vi "Auto Filenames Postprocessing.vi"(8 "Fehler (Eingang)":errorcluster, 9 "active postprocessing index":i32) -> (0 "Fehler (Ausgang)":errorcluster, 1 "active reprocessing index out":i32, 2 "postprocess LIN Filename":string, 3 "postprocess LIN Pfad":path)   [LabVIEW 2020, in "Linearisierung v2.lvlib" / "SpanEinstellungen.lvlib"]
uses:
  SpanEinstellungen.lvlib
  Aktion FGV Post Processing.ctl
  Allgemein/allgemeine Sub-VIs.lvlib
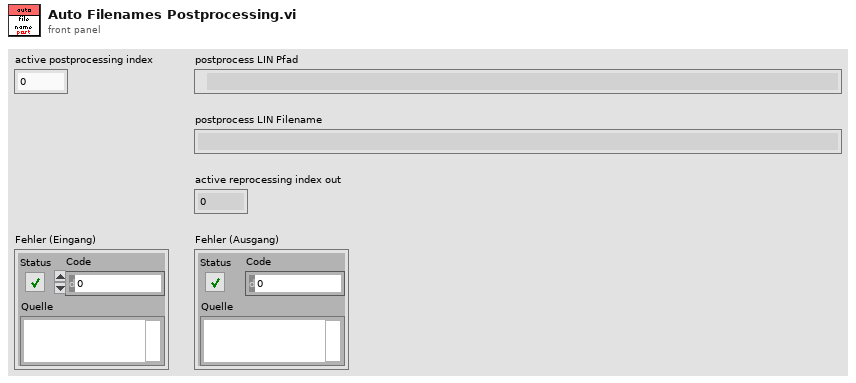
[diagram p1: front panel]
types:
  T1 = typedef "Linearisierung v2.lvlib/SpanEinstellungen.lvlib/Aktion FGV Post Processing.ctl" = enum16{"lesen", "set ref", "init", "reset", "enable", "disable", "filenames", "active", "comp", "filename index", "next", "first", "abort", "show"}
  T2 = typedef "Pfad-Eingabefeld.ctl" = path
  T3 = cluster{"active SPAN Idx":i32, "Pfad .LIN Datei":T2}[]
  T4 = cluster{"active SPAN Idx":i32, "Pfad .LIN Datei":T2}
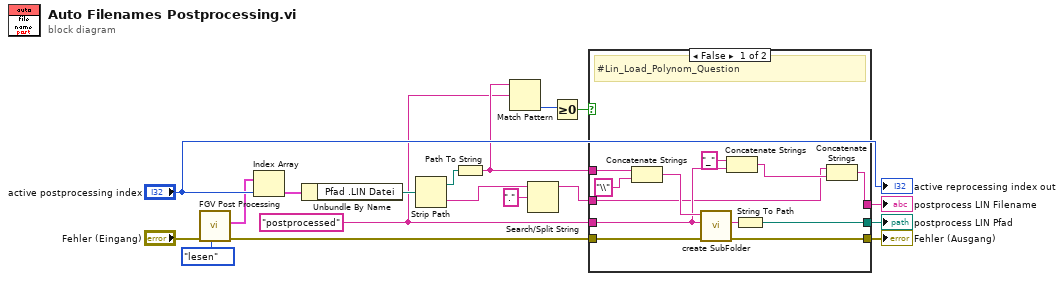
[diagram p0: block diagram]
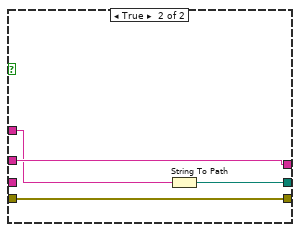
[diagram p2: hidden frame]
diagram:
  w6 = "postprocessed" ("String")
  n1 = call "FGV Post Processing.vi"("Aktion"=Aktion_FGV_Post_Processing."lesen", "error in (no error)"="Fehler (Eingang)") -> ("error out"=w9:errorcluster, "filenemas Cluster Array"=w15:T3)  [unwired: 6 in, 2 out]
  n2 = Index Array(array=w15, index="active postprocessing index") -> (element=w14:T4)
  n3 = Unbundle By Name(w14) -> ("Pfad .LIN Datei"=w13:T2)
  n4 = Strip Path(path=w13) -> (stripped path=w12:path, name=w2:string)
  n5 = Path To String(path=w12) -> (string=w7:string)
  n6 = Match Pattern(string=w7, regular expression=w6) -> (offset past match=w5:i32)  [unwired: 1 in, 3 out]
  n7 = Search/Split String(string=w2, search string/char (-)="." ("Such-String/-Zeichen (-)")) -> (substring before match=w1:string)  [unwired: 1 in, 2 out]
  n8 = Greater Or Equal To 0?(x=w5) -> (x >= 0?=w4:bool)
  n9 = case shown="False" w4 {
    tunnel: [w30 w33] -> w18
    tunnel: [w26 w31] -> w11
    tunnel: w9 -> [w25 w33]
    tunnel: w1 -> [w19 w34]
    tunnel: [w24 w34] -> w8
    tunnel: w7 -> [w21 w32]
    tunnel: w6 -> [w20 _]
    frame False {
      # "#Lin_Load_Polynom_Question"
      n10 = Concatenate Strings(w21, "\\" ("String")) -> (w28:string)
      n11 = call "create SubFolder.vi"("Fehler (Eingang)"=w25, "Ordner"=w20, "Pfad"=w28) -> ("Fehler (Ausgang)"=w30:errorcluster, "SubOrdner"=w29:string)  [unwired: 6 in, 1 out]
      n12 = Concatenate Strings("_" ("String"), w20) -> (w23:string)
      n13 = String To Path(string=w29) -> (path=w26:path)
      n14 = Concatenate Strings(w19, w23) -> (w24:string)
    }
    frame True {
      n15 = String To Path(string=w32) -> (path=w31:path)
    }
  }
  "Fehler (Ausgang)" <- w18
  "postprocess LIN Pfad" <- w11
  "postprocess LIN Filename" <- w8
  "active reprocessing index out" <- "active postprocessing index"
